vi "UpdateTiming.vi"(8 "Timing Plot":refnum<vi>, 11 "TimingPlotData":T1[](array[typedef])) -> ()   [LabVIEW 2013]
uses:
  Controls/TimingPlotData.ctl
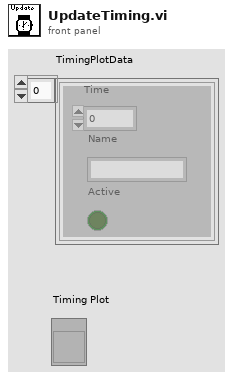
[diagram p1: front panel]
types:
  T1 = typedef "TimingPlotData.ctl" = cluster{"Time":dbl, "Name":string, "Active":bool}
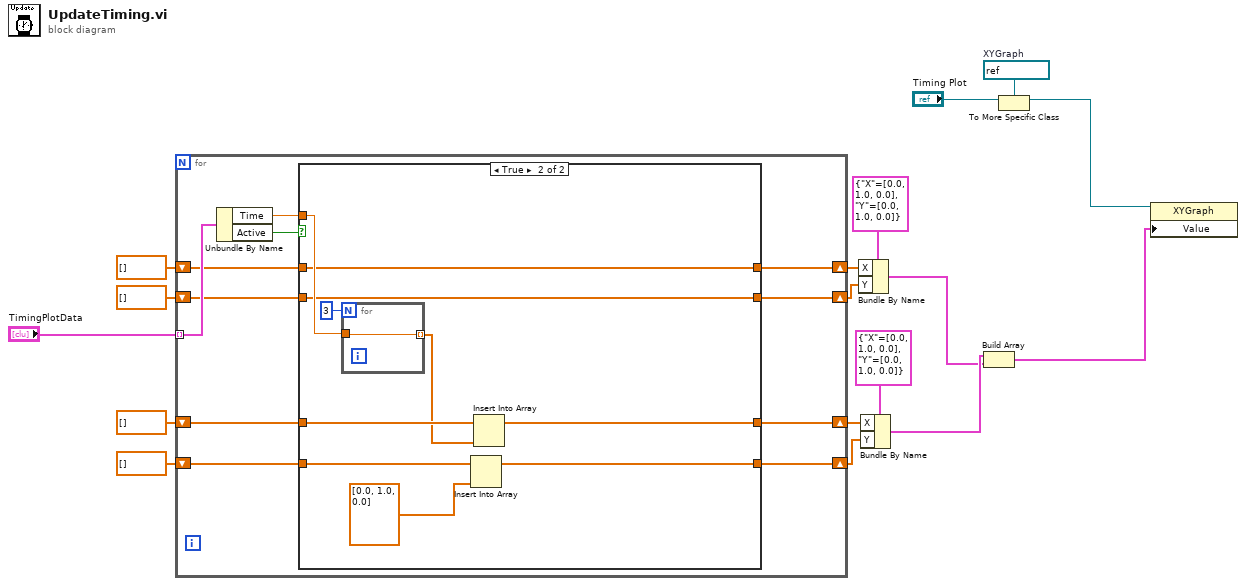
[diagram p0: block diagram]
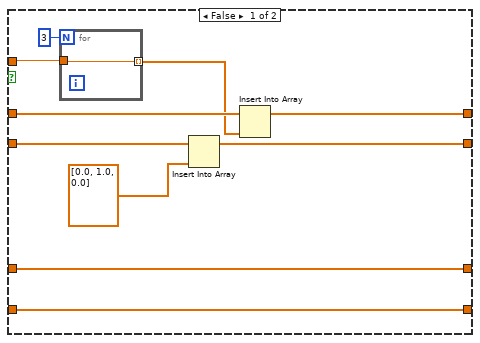
[diagram p2: hidden frame]
diagram:
  w17 = refnum<vi> refnum  # XYGraph
  n1 = for {
    tunnel: "TimingPlotData" -> [w28] mode=indexing
    shift-right: [w23] -> w8
    shift-left: dbl[] [] -> [w20]
    shift-right: [w22] -> w7
    shift-left: dbl[] [] -> [w21]
    shift-right: [w25] -> w11
    shift-left: dbl[] [] -> [w19]
    shift-right: [w24] -> w10
    shift-left: dbl[] [] -> [w18]
    n2 = Unbundle By Name(w28) -> ("Time"=w27:dbl, "Active"=w26:bool)
    n3 = case shown="True" w26 {
      tunnel: w27 -> [w37 w48]
      tunnel: [w31 w41] -> w25
      tunnel: [w33 w40] -> w24
      tunnel: [w35 w46] -> w23
      tunnel: [w36 w43] -> w22
      tunnel: w21 -> [w36 w44]
      tunnel: w20 -> [w35 w47]
      tunnel: w19 -> [w30 w41]
      tunnel: w18 -> [w34 w40]
      frame False {
        n4 = for {
          N: 3 -> [_]
          tunnel: [w39] -> w29 mode=indexing
          tunnel: w37 -> [w39]
        }
        n5 = Insert Into Array(array=w34, new element=dbl[] [0.0, 1.0, 0.0]) -> (w33:dbl[])  [unwired: 1 in]
        n6 = Insert Into Array(array=w30, new element=w29) -> (w31:dbl[])  [unwired: 1 in]
      }
      frame True {
        n7 = for {
          N: 3 -> [_]
          tunnel: [w50] -> w42 mode=indexing
          tunnel: w48 -> [w50]
        }
        n8 = Insert Into Array(array=w47, new element=dbl[] [0.0, 1.0, 0.0]) -> (w46:dbl[])  [unwired: 1 in]
        n9 = Insert Into Array(array=w44, new element=w42) -> (w43:dbl[])  [unwired: 1 in]
      }
    }
  }
  n10 = Bundle By Name(cluster=cluster{"X":dbl[], "Y":dbl[]} {"X"=[0.0, 1.0, 0.0], "Y"=[0.0, 1.0, 0.0]}, "X"=w11, "Y"=w10) -> (w1:cluster{"X":dbl[], "Y":dbl[]})
  n11 = Bundle By Name(cluster=cluster{"X":dbl[], "Y":dbl[]} {"X"=[0.0, 1.0, 0.0], "Y"=[0.0, 1.0, 0.0]}, "X"=w7, "Y"=w8) -> (w2:cluster{"X":dbl[], "Y":dbl[]})
  n12 = Build Array(w2, w1) -> (w13:cluster{"X":dbl[], "Y":dbl[]}[])
  n13 = To More Specific Class(target class=w17, reference="Timing Plot") -> (specific class reference=w15:refnum<vi>)  [unwired: 1 in, 1 out]
  n14 = property class="XYGraph"(reference=w15, "Value"=w13) -> ()  [unwired: 1 in, 2 out]
